vi "Telop Bo Peep.vi"(8 "Safety Lock On":bool, 9 "Turn off vacuum pump and bo peep in":bool, 10 "Turn on vacuum pump and bo peep out":bool, 11 "Safety Lock Off":bool) -> ()   [LabVIEW 2014]
uses:
  <vilib>/Rock Robotics/WPI/Solenoid/WPI_SolenoidValue.ctl
  Robot Global Data.vi
  <vilib>/Rock Robotics/WPI/Solenoid/WPI_SolenoidSetEnum.vi
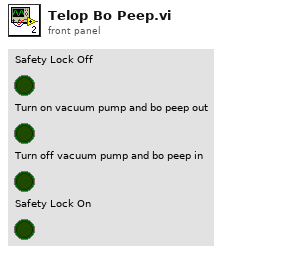
[diagram p1: front panel]
types:
  T1 = typedef "WPI_ServoDeviceRef.ctl" = cluster{"DeviceStatus":errorcluster, "Controller":T2, "PWM Channel":T3, "DeadBand":T4}
  T2 = typedef "FPGA_TypedefDigitalModule.ctl" = enum16{"Controller 1"}
  T3 = typedef "FPGA_DIOPWMChannel.ctl" = enum8{"PWM 0", "PWM 1", "PWM 2", "PWM 3", "PWM 4", "PWM 5", "PWM 6", "PWM 7", "PWM 8", "PWM 9", "PWM MXP 0", "PWM MXP 1", "PWM MXP 2", "PWM MXP 3", "PWM MXP 4", "PWM MXP 5", "PWM MXP 6", "PWM MXP 7", "PWM MXP 8", "PWM MXP 9", "Invalid"}
  T4 = typedef "WPI_PWMDeadband.ctl" = cluster{"Name":string, "maxPositivePwm":i32, "minPositivePwm":i32, "centerPwm":i32, "maxNegativePwm":i32, "minNegativePwm":i32, "angularRange":u16}
  T5 = cluster{"Turn off vacuum pump and bo peep in":bool, bool, bool}
  T6 = typedef "WPI_SolenoidValue.ctl" = enum16{"Off", "On", "Forward", "Reverse"}
  T7 = typedef "WPI_SolenoidDevRef.ctl" = cluster{"DevStatus":errorcluster, "Pneumatics Control Module":u8, "Forward Solenoid Channel":T8, "Reverse Solenoid Channel":T8}
  T8 = typedef "WPI_SolenoidChannel.ctl" = enum8{"Solenoid 0", "Solenoid 1", "Solenoid 2", "Solenoid 3", "Solenoid 4", "Solenoid 5", "Solenoid 6", "Solenoid 7", "Invalid"}
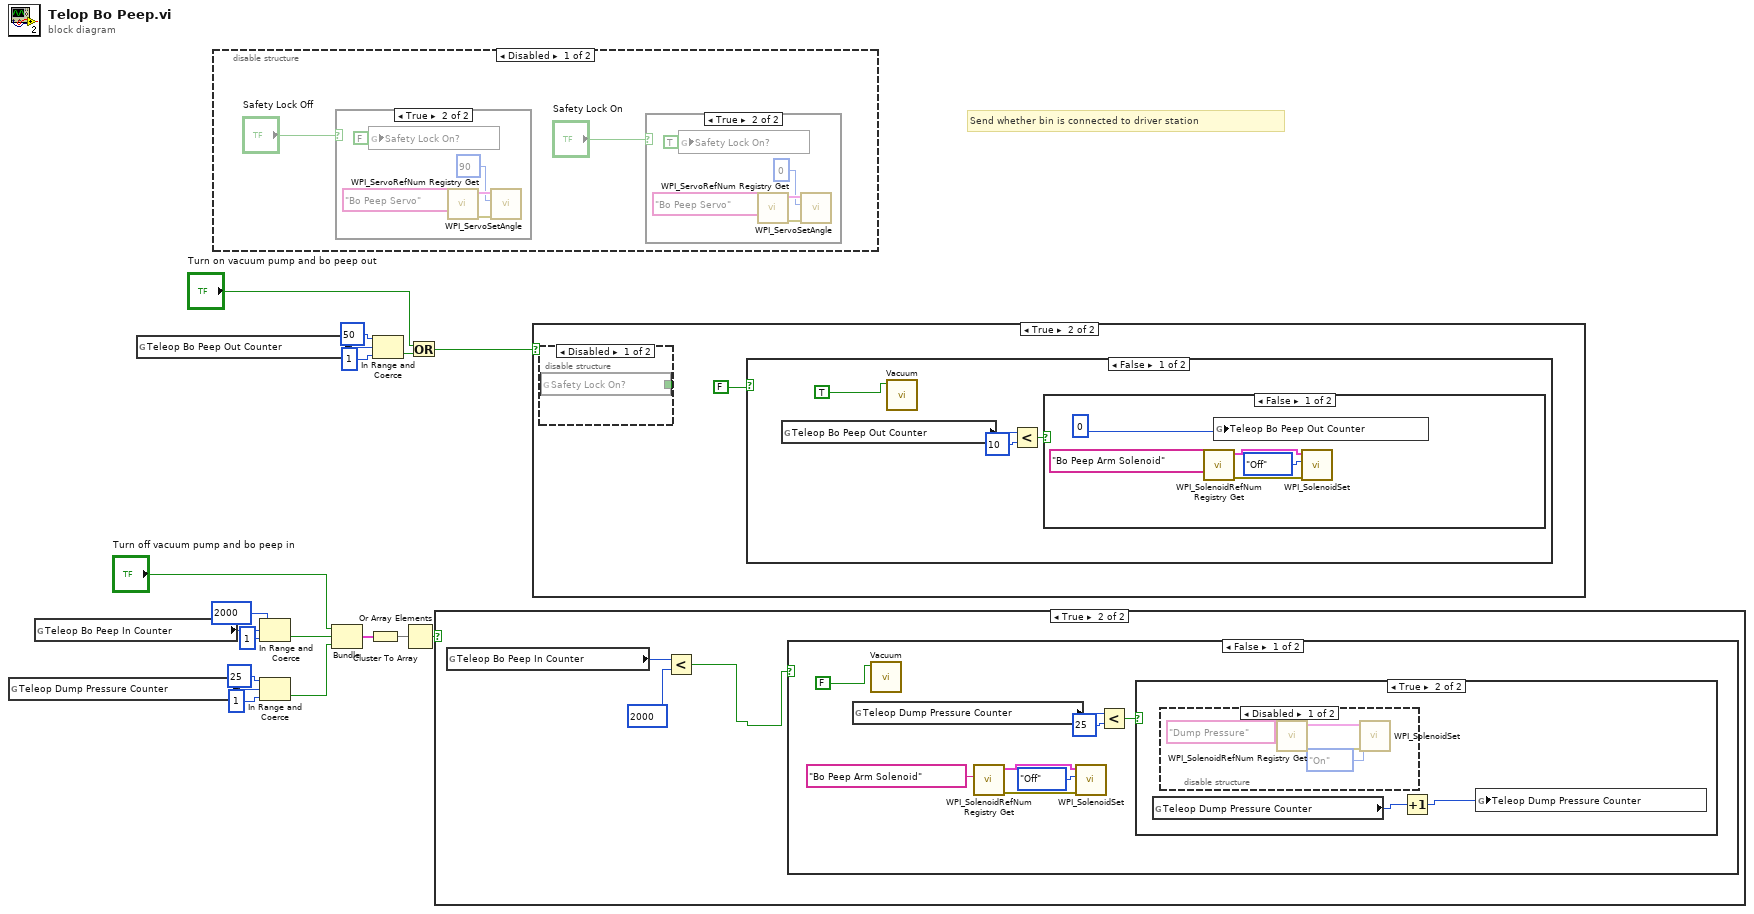
[diagram p0: block diagram]
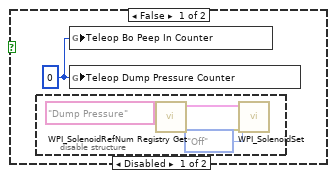
[diagram p6: hidden frame]
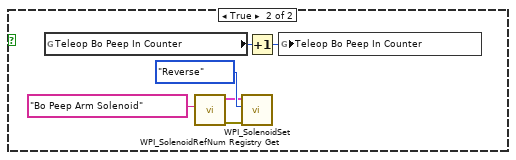
[diagram p9: hidden frame]
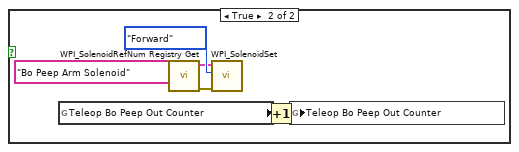
[diagram p12: hidden frame]
diagram:
  # "Send whether bin is connected to driver station"
  n1 = global read "Robot Global Data.vi" "Teleop Dump Pressure Counter"() -> (w9:i8)
  n2 = global read "Robot Global Data.vi" "Teleop Bo Peep In Counter"() -> (w12:u64)
  n3 = global read "Robot Global Data.vi" "Teleop Bo Peep Out Counter"() -> (w16:i8)
  n4 = disable-structure shown="Disabled" {
    frame Disabled {
      n5 = case shown="True" "Safety Lock Off" {
        frame False {
        }
        frame True {
          n6 = global write "Robot Global Data.vi" "Safety Lock On?"(FALSE ("Safety Lock On?")) -> ()
          n7 = call <vilib>:"WPI_ServoRefNum Registry Get.vi"("refnum name"="Bo Peep Servo") -> ("error out"=w29:errorcluster, "ServoDeviceRef"=w28:T1)  [unwired: 9 in]
          n8 = call <vilib>:"WPI_ServoSetAngle.vi"("error in (no error)"=w29, "Angle"=90, "ServoDeviceRef"=w28) -> ()  [unwired: 7 in, 2 out]
        }
      }
      n9 = case shown="True" "Safety Lock On" {
        frame False {
        }
        frame True {
          n10 = global write "Robot Global Data.vi" "Safety Lock On?"(TRUE ("Safety Lock On?")) -> ()
          n11 = call <vilib>:"WPI_ServoRefNum Registry Get.vi"("refnum name"="Bo Peep Servo") -> ("error out"=w24:errorcluster, "ServoDeviceRef"=w23:T1)  [unwired: 9 in]
          n12 = call <vilib>:"WPI_ServoSetAngle.vi"("error in (no error)"=w24, "Angle"=0, "ServoDeviceRef"=w23) -> ()  [unwired: 7 in, 2 out]
        }
      }
    }
    frame Enabled {
    }
  }
  n13 = In Range and Coerce(upper limit=u64 2000, x=w12, lower limit=u64 1) -> (In Range?=w3:bool)  [unwired: 1 out]
  n14 = In Range and Coerce(upper limit=i8 25, x=w9, lower limit=i8 1) -> (In Range?=w8:bool)  [unwired: 1 out]
  n15 = Bundle("Turn off vacuum pump and bo peep in"="Turn off vacuum pump and bo peep in", w3, w8) -> (w7:T5)  [unwired: 1 in]
  n16 = Cluster To Array(cluster=w7) -> (array=w6:bool[])
  n17 = In Range and Coerce(upper limit=i8 50, x=w16, lower limit=i8 1) -> (In Range?=w17:bool)  [unwired: 1 out]
  n18 = Or Array Elements(Boolean array=w6) -> (logical OR=w5:bool)
  n19 = Or(x="Turn on vacuum pump and bo peep out", y=w17) -> (x .or. y?=w13:bool)
  n20 = case shown="True" w5 {
    frame False {
    }
    frame True {
      n21 = global read "Robot Global Data.vi" "Teleop Bo Peep In Counter"() -> (w33:u64)
      n22 = Less?(x=w33, y=u64 2000) -> (x < y?=w32:bool)
      n23 = case shown="False" w32 {
        frame False {
          n24 = global read "Robot Global Data.vi" "Teleop Dump Pressure Counter"() -> (w36:i8)
          n25 = call "Vacuum.vi"("Vacuum State"=FALSE) -> ()  [unwired: 9 in, 1 out]
          n26 = call <vilib>:"WPI_SolenoidRefNum Registry Get.vi"("refnum name"="Bo Peep Arm Solenoid") -> ("error out"=w39:errorcluster, "SolenoidDevRef"=w40:T7)  [unwired: 9 in]
          n27 = call-poly <vilib>:"WPI_SolenoidSet.vi"("error in (no error)"=w39, "Value"=WPI_SolenoidValue."Off", "SolenoidDevRef"=w40) -> ()  [unwired: 7 in, 2 out]
          n28 = Less?(x=w36, y=i8 25) -> (x < y?=w35:bool)
          n29 = case shown="True" w35 {
            frame False {
              w42 = i8 0 ("Teleop Bo Peep Out Counter")
              n30 = disable-structure shown="Disabled" {
                frame Disabled {
                  n31 = call <vilib>:"WPI_SolenoidRefNum Registry Get.vi"("refnum name"="Dump Pressure") -> ("error out"=w46:errorcluster, "SolenoidDevRef"=w44:T7)  [unwired: 9 in]
                  n32 = call-poly <vilib>:"WPI_SolenoidSet.vi"("error in (no error)"=w46, "Value"=WPI_SolenoidValue."Off", "SolenoidDevRef"=w44) -> ()  [unwired: 7 in, 2 out]
                }
                frame Enabled {
                }
              }
              n33 = global write "Robot Global Data.vi" "Teleop Bo Peep In Counter"(w42) -> ()
              n34 = global write "Robot Global Data.vi" "Teleop Dump Pressure Counter"(w42) -> ()
            }
            frame True {
              n35 = global read "Robot Global Data.vi" "Teleop Dump Pressure Counter"() -> (w48:i8)
              n36 = disable-structure shown="Disabled" {
                frame Disabled {
                  n37 = call <vilib>:"WPI_SolenoidRefNum Registry Get.vi"("refnum name"="Dump Pressure") -> ("error out"=w52:errorcluster, "SolenoidDevRef"=w50:T7)  [unwired: 9 in]
                  n38 = call-poly <vilib>:"WPI_SolenoidSet.vi"("error in (no error)"=w52, "Value"=WPI_SolenoidValue."On", "SolenoidDevRef"=w50) -> ()  [unwired: 7 in, 2 out]
                }
                frame Enabled {
                }
              }
              n39 = Increment(x=w48) -> (x+1=w47:i8)
              n40 = global write "Robot Global Data.vi" "Teleop Dump Pressure Counter"(w47) -> ()
            }
          }
        }
        frame True {
          n41 = global read "Robot Global Data.vi" "Teleop Bo Peep In Counter"() -> (w54:u64)
          n42 = call <vilib>:"WPI_SolenoidRefNum Registry Get.vi"("refnum name"="Bo Peep Arm Solenoid") -> ("error out"=w56:errorcluster, "SolenoidDevRef"=w57:T7)  [unwired: 9 in]
          n43 = call-poly <vilib>:"WPI_SolenoidSet.vi"("error in (no error)"=w56, "Value"=WPI_SolenoidValue."Reverse", "SolenoidDevRef"=w57) -> ()  [unwired: 7 in, 2 out]
          n44 = Increment(x=w54) -> (x+1=w53:u64)
          n45 = global write "Robot Global Data.vi" "Teleop Bo Peep In Counter"(w53) -> ()
        }
      }
    }
  }
  n46 = case shown="True" w13 {
    frame False {
    }
    frame True {
      n47 = disable-structure shown="Disabled" {
        disable-tunnel: [w60 _] -> _
        frame Disabled {
          n48 = global read "Robot Global Data.vi" "Safety Lock On?"() -> (w60:bool)
        }
        frame Enabled {
        }
      }
      n49 = case shown="False" FALSE {
        frame False {
          n50 = global read "Robot Global Data.vi" "Teleop Bo Peep Out Counter"() -> (w64:i8)
          n51 = call "Vacuum.vi"("Vacuum State"=TRUE) -> ()  [unwired: 9 in, 1 out]
          n52 = Less?(x=w64, y=i8 10) -> (x < y?=w63:bool)
          n53 = case shown="False" w63 {
            frame False {
              n54 = call <vilib>:"WPI_SolenoidRefNum Registry Get.vi"("refnum name"="Bo Peep Arm Solenoid") -> ("error out"=w67:errorcluster, "SolenoidDevRef"=w68:T7)  [unwired: 9 in]
              n55 = global write "Robot Global Data.vi" "Teleop Bo Peep Out Counter"(i8 0 ("Teleop Bo Peep Out Counter")) -> ()
              n56 = call-poly <vilib>:"WPI_SolenoidSet.vi"("error in (no error)"=w67, "Value"=WPI_SolenoidValue."Off", "SolenoidDevRef"=w68) -> ()  [unwired: 7 in, 2 out]
            }
            frame True {
              n57 = global read "Robot Global Data.vi" "Teleop Bo Peep Out Counter"() -> (w71:i8)
              n58 = call <vilib>:"WPI_SolenoidRefNum Registry Get.vi"("refnum name"="Bo Peep Arm Solenoid") -> ("error out"=w73:errorcluster, "SolenoidDevRef"=w74:T7)  [unwired: 9 in]
              n59 = call-poly <vilib>:"WPI_SolenoidSet.vi"("error in (no error)"=w73, "Value"=WPI_SolenoidValue."Forward", "SolenoidDevRef"=w74) -> ()  [unwired: 7 in, 2 out]
              n60 = Increment(x=w71) -> (x+1=w70:i8)
              n61 = global write "Robot Global Data.vi" "Teleop Bo Peep Out Counter"(w70) -> ()
            }
          }
        }
        frame True {
        }
      }
    }
  }
